vi "Build File Reports.vi"(0 "directory info in":T1={"target dir"=path "C:/ADIBitbucket/nists19.0_templateproject/Code Modules/Common/Instrument Control/DCPower", "output dir"={"base dir"=path "../docs", "image dir"=path "../docs", "html dir"=path "../docs", "md dir"=path "../docs"}, "folder names"=[], "filenames"=[]}, 11 "error in":errorcluster) -> (4 "directory info out":T1={"target dir"=path "C:/ADIBitbucket/nists19.0_templateproject/Code Modules/Common/Instrument Control/DCPower", "output dir"={"base dir"=path "../docs", "image dir"=path "../docs", "html dir"=path "../docs", "md dir"=path "../docs"}, "folder names"=[], "filenames"=[]}, 15 "error out":errorcluster)   [LabVIEW 2019, in "MD Generator.lvlib"]
uses:
  MD Generator.lvlib
  Report Path Cluster.ctl
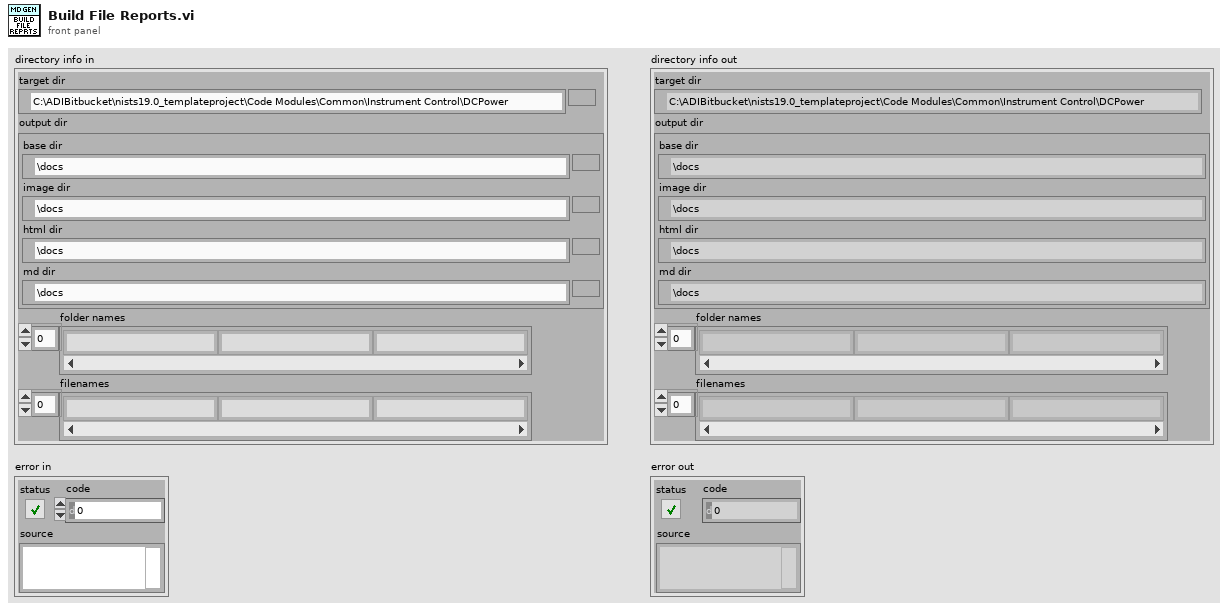
[diagram p1: front panel]
types:
  T1 = typedef "Report Path Cluster.ctl" = cluster{"target dir":path, "output dir":cluster{"base dir":path, "image dir":path, "html dir":path, "md dir":path}, "folder names":string[], "filenames":string[]}
  T2 = enum16{"open", "replace", "create", "open or create", "replace or create", "replace or create with confirmation"}
  T3 = enum32{"Custom", "Standard", "Using Panel", "Using SubVI", "Complete"}
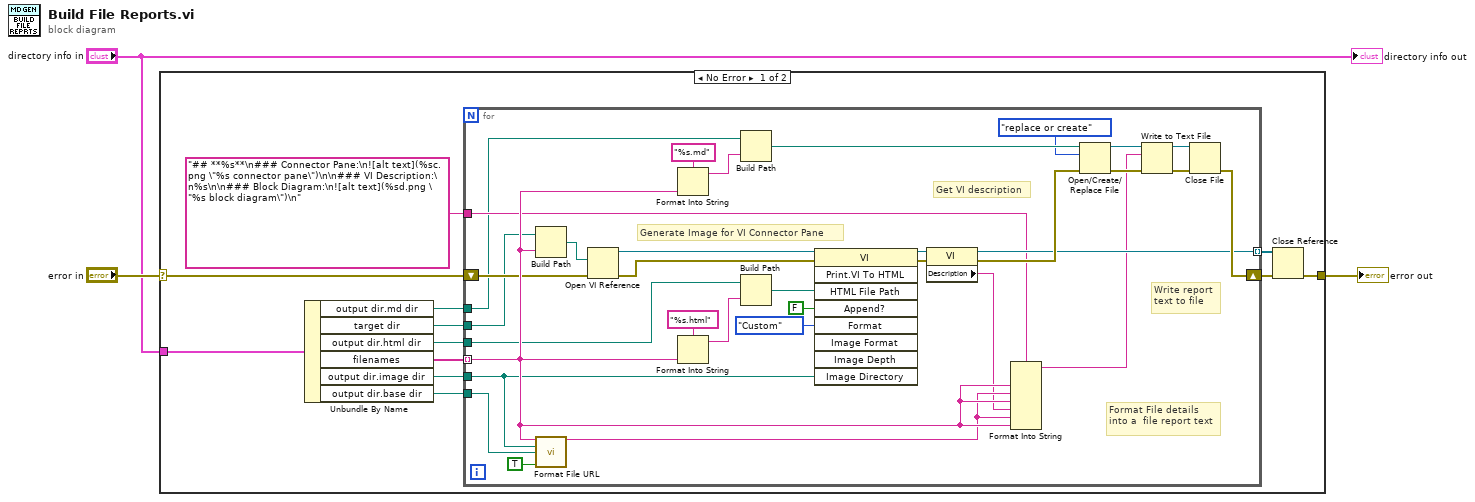
[diagram p0: block diagram]
diagram:
  n1 = case shown="No Error" "error in" {
    selector: "error in" -> [w12 w49]
    tunnel: [w11 w49] -> w2
    tunnel: "directory info in" -> [w15 _]
    frame No Error {
      n2 = Unbundle By Name(w15) -> ("output dir.md dir"=w5:path, "target dir"=w4:path, "output dir.html dir"=w7:path, "filenames"=w8:string[], "output dir.image dir"=w6:path, "output dir.base dir"=w10:path)
      n3 = for {
        shift-right: [w47] -> w13
        shift-left: w12 -> [w43]
        tunnel: [w42] -> w14 mode=indexing
        tunnel: w10 -> [w28]
        tunnel: w8 -> [w48] mode=indexing
        tunnel: "## **%s**\n### Connector Pane:\n![alt text](%sc.png \"%s connector pane\")\n\n### VI Description:\n%s\n\n### Block Diagram:\n![alt text](%sd.png \"%s block diagram\")\n" ("format string") -> [w33]
        tunnel: w7 -> [w27]
        tunnel: w5 -> [w20]
        tunnel: w6 -> [w18]
        tunnel: w4 -> [w17]
        # "Get VI description"
        # "Generate Image for VI Connector Pane"
        # "Write report text to file"
        # "Format File details into a  file report text"
        n4 = Build Path(base path=w17, name or relative path=w48) -> (appended path=w22:path)
        n5 = call "Format File URL.vi"("file name"=w48, "file dir"=w18, "base dir"=w28, "Use HTML Space Formating (%20)"=TRUE) -> ("image URL string"=w29:string)  [unwired: 11 in]
        n6 = Open VI Reference(vi path=w22, error in (no error)=w43) -> (vi reference=w39:refnum<vi>, error out=w41:errorcluster)  [unwired: 4 in]
        n7 = Format Into String(format string="%s.md", w48) -> (resulting string=w23:string)  [unwired: 2 in, 1 out]
        n8 = Format Into String(format string="%s.html", w48) -> (resulting string=w34:string)  [unwired: 2 in, 1 out]
        n9 = Build Path(base path=w20, name or relative path=w23) -> (appended path=w24:path)
        n10 = Build Path(base path=w27, name or relative path=w34) -> (appended path=w35:path)
        n11 = invoke class="VI" method="Print.VI To HTML"(reference=w39, error in=w41, "HTML File Path"=w35, "Append?"=FALSE, "Format"=T3."Custom", "Image Directory"=w18) -> (reference out=w38:refnum<vi>, error out=w40:errorcluster)  [unwired: 3 in, 7 out]
        n12 = property class="VI"(reference=w38, error in=w40) -> (reference out=w42:refnum<vi>, error out=w46:errorcluster, "Description"=w21:string)
        n13 = Format Into String(format string=w33, w48, w29, w48, w21, w29, w48) -> (resulting string=w32:string)  [unwired: 2 in, 1 out]
        n14 = Open/Create/Replace File(file path (use dialog)=w24, error in=w46, operation (0:open)=T2."replace or create") -> (refnum out=w44:refnum<file>, error out=w45:errorcluster)  [unwired: 3 in, 1 out]
        n15 = Write to Text File(file (use dialog)=w44, text=w32, error in=w45) -> (refnum out=w30:refnum<file>, error out=w31:errorcluster)  [unwired: 1 in, 1 out]
        n16 = Close File(refnum=w30, error in=w31) -> (error out=w47:errorcluster)  [unwired: 1 out]
      }
      n17 = Close Reference(reference=w14, error in (no error)=w13) -> (error out=w11:errorcluster)
    }
    frame Error {
    }
  }
  "error out" <- w2
  "directory info out" <- "directory info in"
